vi "PhotodiodeMeasClient.vi"() -> ()   [LabVIEW 2018]
uses:
  Message.ctl
  States.ctl
  <vilib>/NI/STM/SubVIs/MetaDataElement.ctl
  <vilib>/NI/STM/TCP/TCP Read Options.ctl
  <vilib>/NI/STM/TCP/TCP Write Options.ctl
  <vilib>/NI/STM/TCP/Write Meta Data (TCP Ref).vi
  <vilib>/NI/STM/TCP/Get Connection Reference (TCP).vi
  <vilib>/NI/STM/TCP/Write Meta Data (TCP Clst).vi
  <vilib>/NI/STM/TCP/Write Message (TCP).vi
  <vilib>/NI/STM/TCP/Read Message (TCP).vi
  <vilib>/NI/STM/NI STM.lvlib
panel:
  in  "Export path":path=path "C:/temp/result.csv"
  in  "Export":bool
  in  "Delete":bool
  out "Data":i32[](listbox) caption="Measured values"
  out "Unfiltered [count]":u16
  out "B [count]":u16
  out "G [count]":u16
  out "R [count]":u16
  in  "Server IP":string="172.22.11.2"
  in  "Measure":bool
  in  "Stop Button":bool
  in  "LED_3_PWM [%]":u8(slide) scale=0.0..100.0
  in  "LED_2_PWM [%]":u8(slide) scale=0.0..100.0
  in  "LED_1_PWM [%]":u8(slide) scale=0.0..100.0
  # "Controls:\nLED_1_PWM - Set the PWM value of LED_1 \nLED_2_PWM - Set the PWM value of LED_2\nLED_3_PWM - Set the PWM value of LED_3\n\nIndicators:\nR - Last measured red value of the sensor\nG - Last measured green value of the sensor\nB - Last measured blue value of the sensor\nUnfiltered - Last clear value of the sensor\nMeasured Values - Table with the values\n\nButtons:\nMeasure - Get the sensor values\nStop - Stop the program \nDelete - Delete the values from table\nSave  - Save the table in CSV"
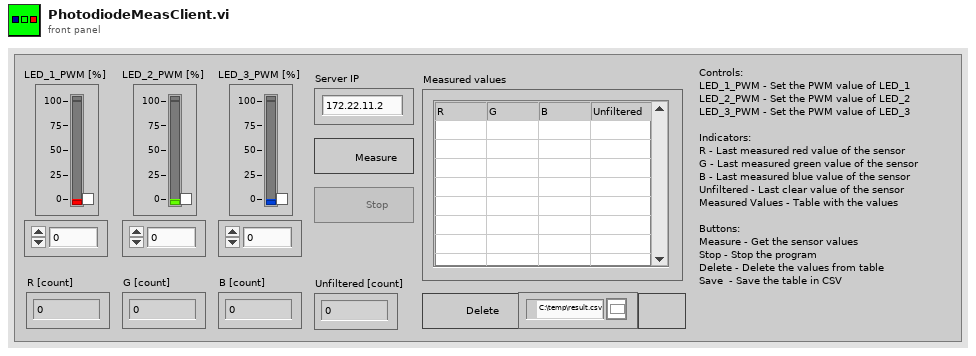
[diagram p1: front panel]
types:
  T1 = typedef "NI STM.lvlib/MetaDataElement.ctl" = string
  T2 = typedef "Message.ctl" = cluster{"States":T3, "Data":variant}
  T3 = typedef "States.ctl" = enum16{"Set LEDs", "Measure", "Exit"}
  T4 = typedef "NI STM.lvlib/TCP Connection Info.ctl" = cluster{"connection ID":refnum<k5>, "meta data":T1[]}
  T5 = typedef "NI STM.lvlib/TCP Read Options.ctl" = cluster{"ignore timeout error":bool, "timeout ms (1000)":i32}
  T6 = typedef "NI STM.lvlib/TCP Write Options.ctl" = cluster{"ignore timeout error":bool, "timeout ms (1000)":i32}
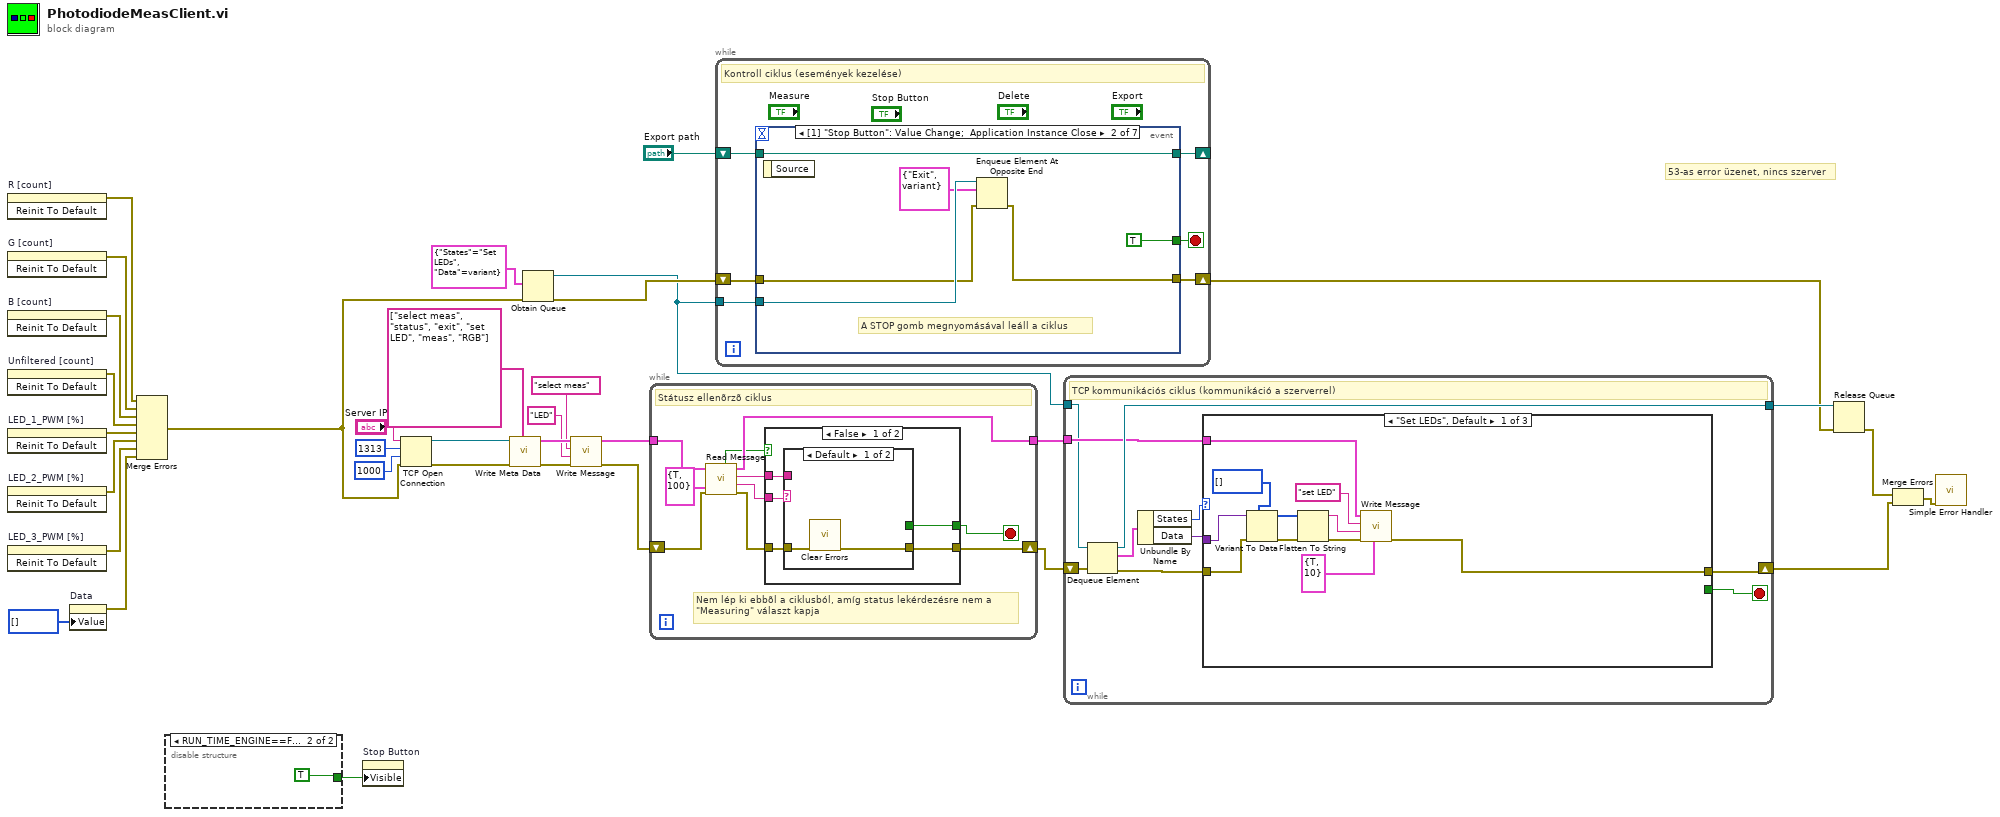
[diagram p0: block diagram]
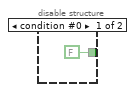
[diagram p2: hidden frame]
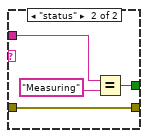
[diagram p3: hidden frame]
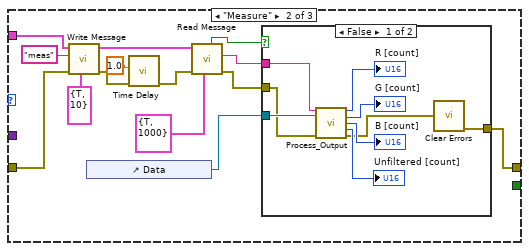
[diagram p5: hidden frame]
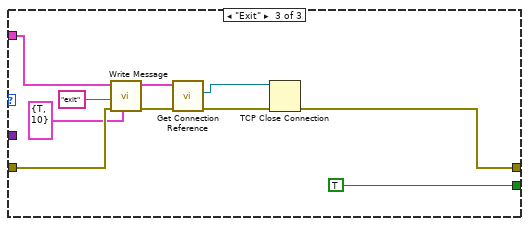
[diagram p7: hidden frame]
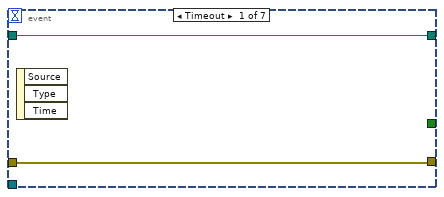
[diagram p8: hidden frame]
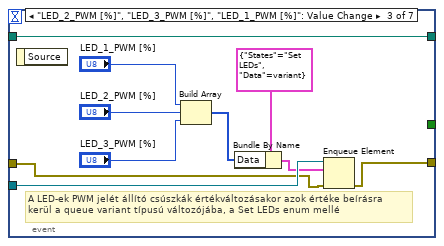
[diagram p9: hidden frame]
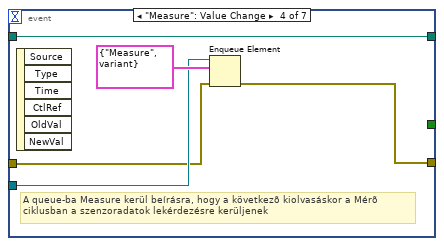
[diagram p10: hidden frame]
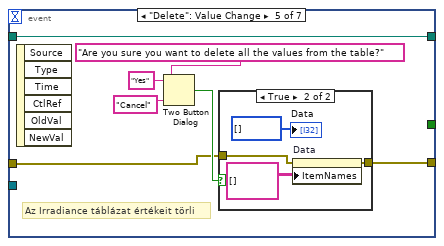
[diagram p11: hidden frame]
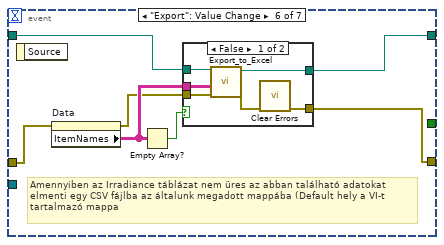
[diagram p13: hidden frame]
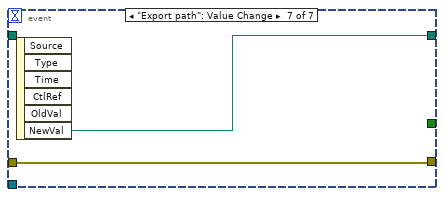
[diagram p15: hidden frame]
diagram:
  # "53-as error üzenet, nincs szerver"
  n1 = invoke on="R [count]" class="DigNum (strict)" method="Reinit To Default"() -> (error out=w13:errorcluster)  [unwired: 3 in, 2 out]
  n2 = invoke on="G [count]" class="DigNum (strict)" method="Reinit To Default"() -> (error out=w12:errorcluster)  [unwired: 3 in, 2 out]
  n3 = invoke on="B [count]" class="DigNum (strict)" method="Reinit To Default"() -> (error out=w11:errorcluster)  [unwired: 3 in, 2 out]
  n4 = invoke on="Unfiltered [count]" class="DigNum (strict)" method="Reinit To Default"() -> (error out=w10:errorcluster)  [unwired: 3 in, 2 out]
  n5 = invoke on="LED_1_PWM [%]" class="Slide (strict)" method="Reinit To Default"() -> (error out=w9:errorcluster)  [unwired: 3 in, 2 out]
  n6 = invoke on="LED_2_PWM [%]" class="Slide (strict)" method="Reinit To Default"() -> (error out=w8:errorcluster)  [unwired: 3 in, 2 out]
  n7 = invoke on="LED_3_PWM [%]" class="Slide (strict)" method="Reinit To Default"() -> (error out=w7:errorcluster)  [unwired: 3 in, 2 out]
  n8 = property on="Data" class="MCListbox (strict)"("Value"=i32[] [] ("Data")) -> (error out=w3:errorcluster)  [unwired: 2 in, 1 out]
  n9 = Merge Errors(w13, w12, w11, w10, w9, w8, w7, w3) -> (w2:errorcluster)
  n10 = disable-structure shown="RUN_TIME_ENGINE==False" {
    disable-tunnel: [FALSE TRUE] -> w1
    frame condition #0 {
    }
    frame condition #1 (active) {
    }
  }
  n11 = property on="Stop Button" class="Bool"("Visible"=w1) -> ()  [unwired: 2 in, 2 out]
  n12 = TCP Open Connection(address="Server IP", remote port or service name=u16 1313, timeout ms (60000)=1000, error in (no error)=w2) -> (connection ID=w31:refnum<k5>, error out=w32:errorcluster)  [unwired: 1 in]
  n13 = call-poly <vilib>:"Write Meta Data.vi"("meta data"=T1[] ["select meas", "status", "exit", "set LED", "meas", "RGB"], "error in"=w32, "connection ID"=w31) -> ("error out"=w26:errorcluster, "connection info out"=w25:T4)  [unwired: 7 in]
  n14 = Obtain Queue(element data type=T2 {"States"=enum."Set LEDs", "Data"=variant} ("Message"), error in (no error)=w2) -> (queue out=w6:refnum<queue>, error out=w14:errorcluster)  [unwired: 3 in, 1 out]
  n15 = call-poly <vilib>:"Write Message.vi"("error in"=w26, "data"="LED", "name"="select meas", "connection info in"=w25) -> ("error out"=w18:errorcluster, "connection info out"=w22:T4)  [unwired: 6 in]
  n16 = while {
    tunnel: w22 -> [w46]
    tunnel: [w45] -> w21
    shift-right: [w39] -> w5
    shift-left: w18 -> [w40]
    stop <- w38 stop-if-true
    # "Nem lép ki ebbõl a ciklusból, amíg status lekérdezésre nem a \n\"Measuring\" választ kapja"
    # "Státusz ellenõrzõ ciklus"
    n17 = call-poly <vilib>:"Read Message.vi"("options"=T5 {"ignore timeout error"=TRUE, "timeout ms (1000)"=100}, "error in"=w40, "connection info in"=w46) -> ("error out"=w41:errorcluster, "name"=w42:T1, "data string"=w43:string, "connection info out"=w45:T4, "timed out?"=w37:bool)  [unwired: 3 in, 1 out]
    n18 = case shown="False" w37 {
      tunnel: w43 -> [w50 _]
      tunnel: w42 -> [w49 _]
      tunnel: [w51 _] -> w38
      tunnel: w41 -> [w48 w58]
      tunnel: [w47 w58] -> w39
      frame False {
        n19 = case shown="Default" w49 {
          tunnel: w50 -> [_ w54]
          tunnel: [_ w57] -> w51
          tunnel: w48 -> [w53 w55]
          tunnel: [w52 w55] -> w47
          frame Default {
            n20 = call <vilib>:"Clear Errors.vi"("error in (no error)"=w53) -> ("error out"=w52:errorcluster)  [unwired: 5 in, 1 out]
          }
          frame "status" {
            n21 = Equal?(x=w54, y="Measuring") -> (x = y?=w57:bool)
          }
        }
      }
      frame True {
      }
    }
  }
  n22 = while {
    tunnel: w6 -> [w63]
    shift-right: [w62] -> _
    shift-left: "Export path" -> [w61]
    shift-right: [w60] -> w17
    shift-left: w14 -> [w59]
    stop <- w64 stop-if-true
    # "Kontroll ciklus (események kezelése)"
    n23 = event shown="[1] \"Stop Button\": Value Change;  Application Instance Close" {
      selector: _ -> [_ _ _ _ _ _ _]
      dyn-events: _ -> [_ _ _ _ _ _ _]
      timeout: _ -> [_ _ _ _ _ _ _]
      tunnel: [_ TRUE _ _ _ _ _] -> w64
      tunnel: w63 -> [_ w72 w81 w86 _ _ _]
      tunnel: [w66 w70 w76 w85 w90 w103 w116] -> w62
      tunnel: w61 -> [w66 w70 w76 w85 w90 w104 _]
      tunnel: [w65 w67 w73 w84 w88 w100 w115] -> w60
      tunnel: w59 -> [w65 w68 w74 w83 w89 w101 w115]
      event Timeout {
        n24 = event-data() -> ()  [unwired: 1 in, 3 out]
      }
      event "Stop Button": Value Change; Application Instance Close {
        # "A STOP gomb megnyomásával leáll a ciklus"
        n25 = event-data() -> ()  [unwired: 1 in, 1 out]
        n26 = Enqueue Element At Opposite End(queue=w72, element=T2 {"States"=enum."Exit", "Data"=variant}, error in (no error)=w68) -> (error out=w67:errorcluster)  [unwired: 1 in, 2 out]
      }
      event "LED_2_PWM [%]", "LED_3_PWM [%]", "LED_1_PWM [%]": Value Change {
        # "A LED-ek PWM jelét állító csúszkák értékváltozásakor azok értéke beírásra\nkerül a queue variant típusú változójába, a Set LEDs enum mellé"
        n27 = event-data() -> ()  [unwired: 1 in, 1 out]
        n28 = Build Array("LED_1_PWM [%]", "LED_2_PWM [%]", "LED_3_PWM [%]") -> (w77:u8[])
        n29 = Bundle By Name(cluster=T2 {"States"=enum."Set LEDs", "Data"=variant} ("element"), "Data"=w77) -> (w80:T2)
        n30 = Enqueue Element(queue=w81, element=w80, error in (no error)=w74) -> (error out=w73:errorcluster)  [unwired: 1 in, 2 out]
      }
      event "Measure": Value Change {
        # "A queue-ba Measure kerül beírásra, hogy a következõ kiolvasáskor a Mérõ \nciklusban a szenzoradatok lekérdezésre kerüljenek"
        n31 = event-data() -> ()  [unwired: 1 in, 6 out]
        n32 = Enqueue Element(queue=w86, element=T2 {"States"=enum."Measure", "Data"=variant}, error in (no error)=w83) -> (error out=w84:errorcluster)  [unwired: 1 in, 2 out]
      }
      event "Delete": Value Change {
        # "Az Irradiance táblázat értékeit törli"
        n33 = event-data() -> ()  [unwired: 1 in, 6 out]
        n34 = Two Button Dialog(message="Are you sure you want to delete all the values from the table?", 1:"Cancel" ("F button name (\"Cancel\")"), 2:"Yes" ("T button name (\"OK\")")) -> (T button?=w91:bool)
        n35 = case shown="True" w91 {
          tunnel: w89 -> [w95 w97]
          tunnel: [w95 w96] -> w88
          frame False {
          }
          frame True {
            n36 = property on="Data" class="MCListbox (strict)"(error in=w97, "ItemNames"=string[][] [] ("Item Names")) -> (error out=w96:errorcluster)  [unwired: 1 in, 1 out]
            "Data" <- i32[] [] ("Data")
          }
        }
      }
      event "Export": Value Change {
        # "Amennyiben az Irradiance táblázat nem üres az abban található adatokat\nelmenti egy CSV fájlba az általunk megadott mappába (Default hely a VI-t\ntartalmazó mappa"
        n37 = event-data() -> ()  [unwired: 1 in, 1 out]
        n38 = property on="Data" class="MCListbox (strict)"(error in=w101) -> (error out=w102:errorcluster, "ItemNames"=w105:string[][])  [unwired: 1 in, 1 out]
        n39 = Empty Array?(array=w105) -> (empty?=w106:bool)
        n40 = case shown="False" w106 {
          tunnel: w105 -> [w112 _]
          tunnel: w104 -> [w110 w114]
          tunnel: [w109 w114] -> w103
          tunnel: w102 -> [w108 w113]
          tunnel: [w107 w113] -> w100
          frame False {
            n41 = call "Export_to_Excel.vi"("Error In"=w108, "Incoming data"=w112, "Export path"=w110) -> ("Error Out"=w111:errorcluster, "New path"=w109:path)  [unwired: 3 in]
            n42 = call <vilib>:"Clear Errors.vi"("error in (no error)"=w111) -> ("error out"=w107:errorcluster)  [unwired: 5 in, 1 out]
          }
          frame True {
          }
        }
      }
      event "Export path": Value Change {
        n43 = event-data() -> ("NewVal"=w116:path)  [unwired: 1 in, 5 out]
      }
    }
  }
  n44 = while {
    shift-right: [w121] -> w15
    shift-left: w5 -> [w126]
    tunnel: w21 -> [w119]
    tunnel: [w120] -> w29
    tunnel: w6 -> [w117]
    stop <- w118 stop-if-true
    # "TCP kommunikációs ciklus (kommunikáció a szerverrel)"
    n45 = Dequeue Element(queue=w117, error in (no error)=w126) -> (queue out=w120:refnum<queue>, element=w125:T2, error out=w123:errorcluster)  [unwired: 1 in, 1 out]
    n46 = Unbundle By Name(w125) -> ("States"=w124:T3, "Data"=w122:variant)
    n47 = case shown="\"Set LEDs\", Default" w124 {
      tunnel: [_ _ TRUE] -> w118
      tunnel: w123 -> [w137 w150 w167]
      tunnel: w122 -> [w136 _ _]
      tunnel: [w127 w149 w168] -> w121
      tunnel: w119 -> [w132 w151 w166]
      frame "Set LEDs", Default {
        n48 = Variant To Data(error in=w137, type=u8[] [], Variant=w136) -> (data=w131:u8[], error out=w130:errorcluster)
        n49 = Flatten To String(anything=w131, error in (no error)=w130) -> (data string=w128:string, error out=w129:errorcluster)  [unwired: 2 in, 1 out]
        n50 = call-poly <vilib>:"Write Message.vi"("options"=T6 {"ignore timeout error"=TRUE, "timeout ms (1000)"=10}, "error in"=w129, "data"=w128, "name"="set LED", "connection info in"=w132) -> ("error out"=w127:errorcluster)  [unwired: 5 in, 1 out]
      }
      frame "Measure" {
        n51 = call-poly <vilib>:"Write Message.vi"("options"=T6 {"ignore timeout error"=TRUE, "timeout ms (1000)"=10}, "error in"=w150, "name"="meas", "connection info in"=w151) -> ("error out"=w142:errorcluster, "connection info out"=w139:T4)  [unwired: 6 in]
        n52 = control-ref of="Data"() -> (w138:refnum<vi>)
        n53 = call "Time Delay"("error in (no error)"=w142, "Delay Time (s)"=1.0) -> ("error out"=w141:errorcluster)  [unwired: 9 in]
        n54 = call-poly <vilib>:"Read Message.vi"("options"=T5 {"ignore timeout error"=TRUE, "timeout ms (1000)"=1000}, "error in"=w141, "connection info in"=w139) -> ("error out"=w143:errorcluster, "data string"=w145:string, "timed out?"=w146:bool)  [unwired: 3 in, 3 out]
        n55 = case shown="False" w146 {
          tunnel: w145 -> [w159 _]
          tunnel: w143 -> [w157 w161]
          tunnel: [w160 w161] -> w149
          tunnel: w138 -> [w158 _]
          frame False {
            n56 = call "Process_Output.vi"("Data string"=w159, "Table reference"=w158, "Error In"=w157) -> ("R"=→"R [count]":u16, "G"=→"G [count]":u16, "B"=→"B [count]":u16, "Unfiltered"=→"Unfiltered [count]":u16, "Error Out"=w152:errorcluster)  [unwired: 8 in]
            n57 = call <vilib>:"Clear Errors.vi"("error in (no error)"=w152) -> ("error out"=w160:errorcluster)  [unwired: 5 in, 1 out]
          }
          frame True {
          }
        }
      }
      frame "Exit" {
        n58 = call-poly <vilib>:"Write Message.vi"("options"=T6 {"ignore timeout error"=TRUE, "timeout ms (1000)"=10}, "error in"=w167, "name"="exit", "connection info in"=w166) -> ("error out"=w165:errorcluster, "connection info out"=w164:T4)  [unwired: 6 in]
        n59 = call-poly <vilib>:"Get Connection Reference.vi"("error in"=w165, "connection info in"=w164) -> ("error out"=w170:errorcluster, "connection ID out"=w169:refnum<k5>)  [unwired: 7 in, 1 out]
        n60 = TCP Close Connection(connection ID=w169, error in (no error)=w170) -> (error out=w168:errorcluster)  [unwired: 1 in, 1 out]
      }
    }
  }
  n61 = Release Queue(queue=w29, error in (no error)=w17) -> (error out=w16:errorcluster)  [unwired: 1 in, 2 out]
  n62 = Merge Errors(w16, w15) -> (w28:errorcluster)
  n63 = call <vilib>:"Simple Error Handler.vi"("error in (no error)"=w28) -> ()  [unwired: 4 in, 5 out]
